vi "Get Folder IDs.vi"(6 "OPC UA server":T1, 8 "error in (no error)":errorcluster, 9 "Tx Folder NodeIDs":string[](array[string]), 10 "Rx Folder NodeIDs":string[](array[string]), 11 "Station Actor in":refnum<class "Station Actor.lvclass">) -> (0 "error out":errorcluster, 3 "Station Actor out":refnum<class "Station Actor.lvclass">)   [LabVIEW 2019]
uses:
  Station Actor.lvclass
  C:/Program Files (x86)/National Instruments/LabVIEW 2019/vi.lib/ActorFramework/Actor/Actor.lvclass
  <vilib>/OPCUA/controls/OPC UA Server Refnum.ctl
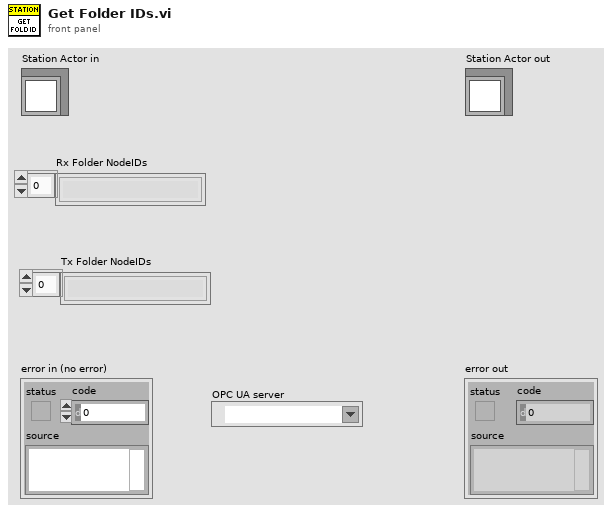
[diagram p1: front panel]
types:
  T1 = typedef "OPC UA Server Refnum.ctl" = refnum<k21>
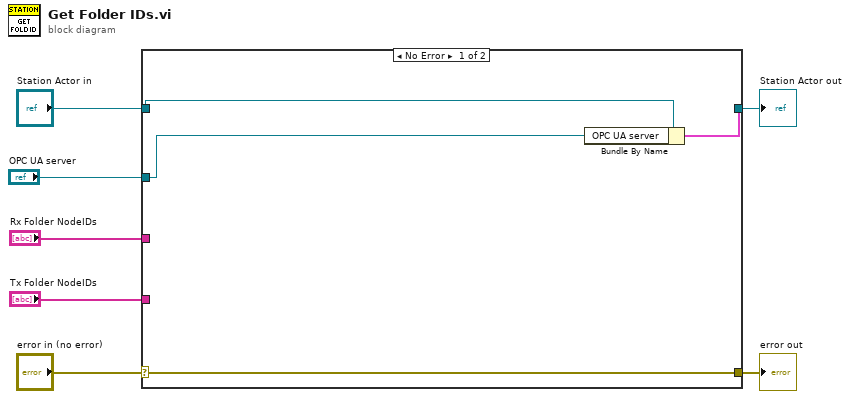
[diagram p0: block diagram]
diagram:
  n1 = case shown="No Error" "error in (no error)" {
    selector: "error in (no error)" -> [w11 w13]
    tunnel: [w11 w13] -> w6
    tunnel: [w8 w12] -> w4
    tunnel: "Station Actor in" -> [w10 w12]
    tunnel: "OPC UA server" -> [w9 _]
    tunnel: "Rx Folder NodeIDs" -> [_ _]
    tunnel: "Tx Folder NodeIDs" -> [_ _]
    frame No Error {
      n2 = Bundle By Name(cluster=w10, "OPC UA server"=w9) -> (w8:cluster{})
    }
    frame Error {
    }
  }
  "error out" <- w6
  "Station Actor out" <- w4
